vi "Deactivate ChnlHW.vi"(8 "error in (no error)":errorcluster, 10 "ChnlName":string, 11 "BME_DG_System in":refnum<class "BME_DG_System.lvclass">) -> (0 "error out":errorcluster, 3 "BME_DG_System out":refnum<class "BME_DG_System.lvclass">)   [LabVIEW 2009, in "POLARIS BME DG.lvlib" / "BME_DG_System.lvclass"]
uses:
  BME_DG_System.lvclass
  BME_DG_Chnl/BME_DG_Chnl.lvclass
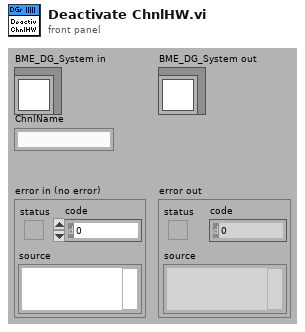
[diagram p1: front panel]
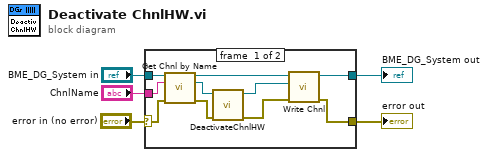
[diagram p0: block diagram]
diagram:
  n1 = case shown="No Error" "error in (no error)" {
    selector: "error in (no error)" -> [w13 w17]
    tunnel: [w10 w17] -> w4
    tunnel: [w11 w16] -> w2
    tunnel: "BME_DG_System in" -> [w15 w16]
    tunnel: "ChnlName" -> [w14 _]
    frame #0 {
      n2 = call "Get Chnl by Name.vi"("BME_DG_System in"=w15, "Chnl Name"=w14, "error in (no error)"=w13) -> ("BME_DG_System out"=w12:refnum<class "BME_DG_System.lvclass">, "BME_DG_Chnl"=w9:refnum<class "BME_DG_Chnl.lvclass">, "error out"=w6:errorcluster)  [unwired: 7 in, 3 out]
      n3 = call-dynamic "DeactivateChnlHW.vi"("error in (no error)"=w6, "BME_DG_Chnl in"=w9) -> ("error out"=w7:errorcluster, "BME_DG_Chnl out"=w8:refnum<class "BME_DG_Chnl.lvclass">)  [unwired: 8 in]
      n4 = call "Write Chnl.vi"("error in (no error)"=w7, "BME_DG_Chnl.lvclass"=w8, "BME_DG_System in"=w12) -> ("error out"=w10:errorcluster, "BME_DG_System out"=w11:refnum<class "BME_DG_System.lvclass">)  [unwired: 7 in]
    }
    frame #1 {
    }
  }
  "error out" <- w4
  "BME_DG_System out" <- w2
